vi "User.Global.vi"() -> ()   [LabVIEW 2016]
uses:
  User.Info.ctl
  User.Level.ctl
panel:
  in  "FilePath":path
  in  "LoginTimeout":dbl format="%#.3g"
  out "Guru TS":timestamp
  out "Guru":bool
  out "Temp Guru":string
  in  "UserLevel":T1
  in  "UserLoggedIn":i32
  in  "Admin Pass":string="9362d067b30452cfb42e081a23b79198"
  in  "Admin User":string="Guru"
  in  "DefaultUser":string="-"
  in  "Users":T2[](array[typedef])
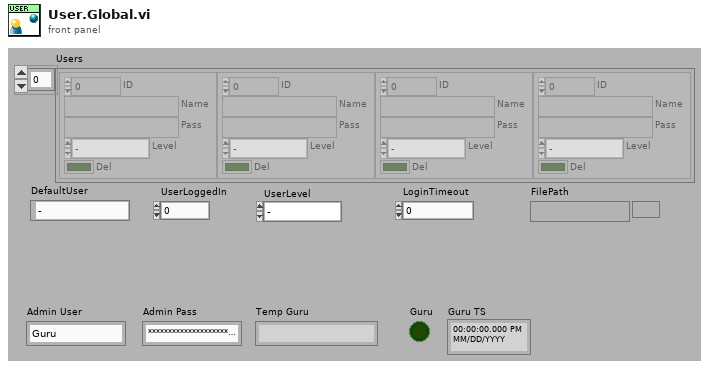
[diagram p1: front panel]
types:
  T1 = typedef "User.Level.ctl" = enum16{"-", "Operator", "Technician", "Administrator"}
  T2 = typedef "User.Info.ctl" = cluster{"ID":i32, "Name":string, "Pass":string, "Level":T1, "Del":bool}
diagram:
